vi "Example.vi"() -> ()   [LabVIEW 2014, in "ND2_Reader_32.lvlib"]
uses:
  ND2_Reader_32.lvlib
panel:
  out "Image":T1(plugin-control)
  out "Avg Frame Process Time":dbl
  in  "stop":bool
  out "Frame Timing":u32(graph)
  out "Process Time":dbl
  in  "FilePath":path=path "C:/Users/VirtualUser/Desktop/EPA Image Processing/test images/150806-005.nd2"
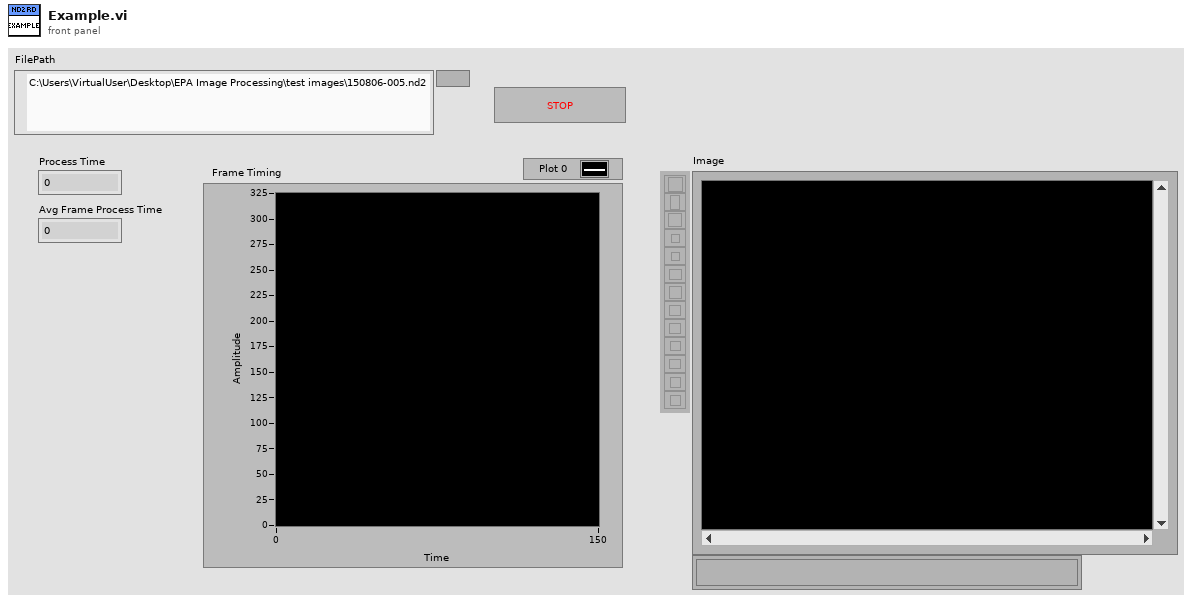
[diagram p1: front panel]
types:
  T1 = typedef "IMAQ Image.ctl" = refnum<image>
  T2 = typedef "cluster_LIMPICTURE.ctl" = cluster{"uiWidth":u32, "uiHeight":u32, "uiBitsPerComp":u32, "uiComponents":u32, "uiWidthBytes":u32, "uiSize":u32, "pImageData":u32}
  T3 = typedef "numeric_LIMFILEHANDLE.ctl" = i32
  T4 = typedef "Image Type" = u32
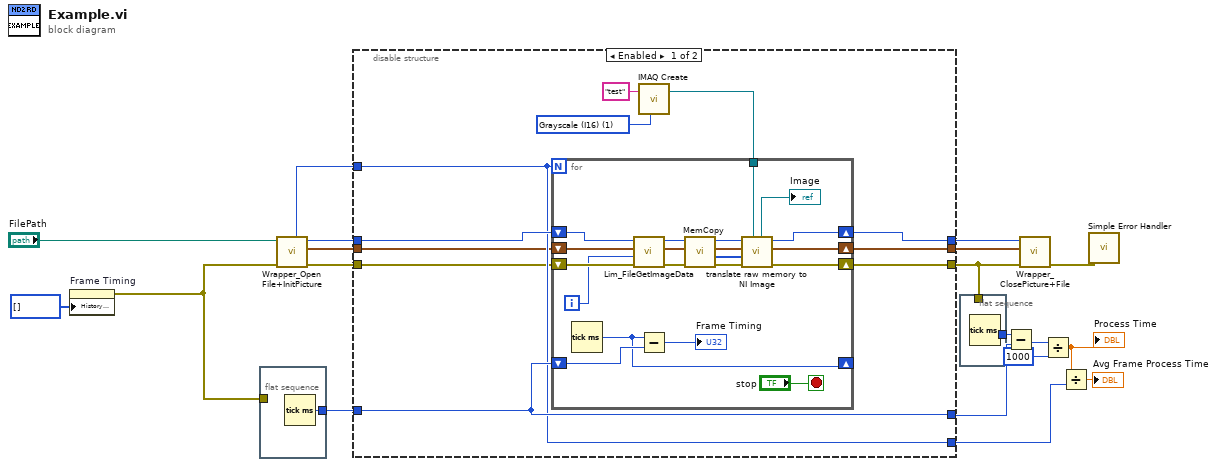
[diagram p0: block diagram]
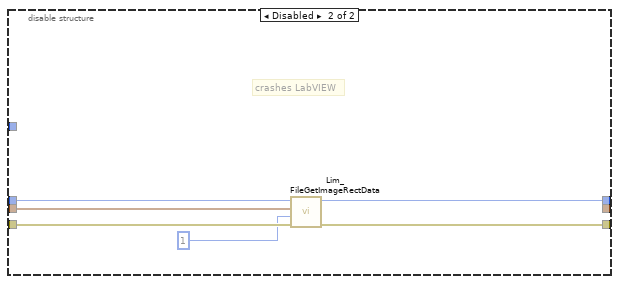
[diagram p2: hidden frame]
diagram:
  n1 = property on="Frame Timing" class="WFChart (strict)"("History Data"=u32[] []) -> (error out=w6:errorcluster)  [unwired: 2 in, 1 out]
  n2 = flat-sequence {
    tunnel: [w20] -> w18
    tunnel: w6 -> [_]
    frame #0 {
      n3 = Tick Count (ms)() -> (millisecond timer value=w20:u32)
    }
  }
  n4 = call "Wrapper_Open File+InitPicture.vi"("error in (no error)"=w6, "FilePath"="FilePath") -> ("error out"=w10:errorcluster, "LIMPICTUREout"=w9:T2, "hFile out"=w8:T3, "N Frames (= uiSequenceCount)"=w5:u32)  [unwired: 6 in]
  n5 = disable-structure shown="Enabled" {
    disable-tunnel: [w22 w55] -> w4
    disable-tunnel: [w23 w56] -> w2
    disable-tunnel: w9 -> [w24 w53]
    disable-tunnel: w8 -> [w27 w57]
    disable-tunnel: w10 -> [w25 w54]
    disable-tunnel: w18 -> [w31 _]
    disable-tunnel: [w31 _] -> w16
    disable-tunnel: [w26 _] -> w12
    disable-tunnel: w5 -> [w26 _]
    disable-tunnel: [w21 _] -> w1
    frame Enabled {
      w29 = T4 1 items=["Grayscale (U8)", "Grayscale (I16)", "Grayscale (SGL)", "Complex (CSG)", "RGB (U32)", "HSL (U32)", "RGB (U64)", "Grayscale (U16)"] ("Image Type")
      n6 = call "IMAQ Create"("Image Name"="test", "Image Type"=w29) -> ("New Image"=w28:T1)  [unwired: 3 in, 1 out]
      n7 = for {
        N: w26 -> [_]
        shift-right: [w43] -> w23
        shift-left: w27 -> [w51]
        shift-right: [w32] -> w21
        shift-left: w24 -> [w50]
        shift-right: [w42] -> w22
        shift-left: w25 -> [w49]
        shift-right: [w46] -> _
        shift-left: w31 -> [w47]
        tunnel: w28 -> [w40]
        i -> [w48]
        stop <- "stop" stop-if-true
        n8 = Tick Count (ms)() -> (millisecond timer value=w46:u32)
        n9 = call "Lim_FileGetImageData.vi"("error in (no error)"=w49, "frameindex"=w48, "LIMPICTURE in"=w50, "hFile in"=w51) -> ("error out"=w45:errorcluster, "LIMPICTURE out"=w33:T2, "hFile out"=w44:T3)  [unwired: 4 in, 1 out]
        n10 = Subtract(x=w46, y=w47) -> (x-y=→"Frame Timing":u32)
        n11 = call "MemCopy.vi"("error in (no error)"=w45, "LIMPICTURE in"=w33, "hFile in"=w44) -> ("error out"=w38:errorcluster, "pBuffer out"=w34:u8[], "LIMPICTURE out"=w35:T2, "hFile out"=w37:T3)  [unwired: 5 in]
        n12 = call "translate raw memory to NI Image.vi"("Image in"=w40, "error in (no error)"=w38, "pBuffer"=w34, "LIMPICTURE in"=w35, "hFile in"=w37) -> ("error out"=w42:errorcluster, "LIMPICTURE out"=w32:T2, "hFile out"=w43:T3, "Image out"=→"Image":T1)  [unwired: 3 in]
      }
    }
    frame Disabled {
      # "crashes LabVIEW"
      n13 = call "Lim_FileGetImageRectData.vi"("error in (no error)"=w54, "frameindex"=u32 1, "LIMATTRIBUTES"=w53, "hFile in"=w57) -> ("error out"=w55:errorcluster, "hFile out"=w56:T3)  [unwired: 5 in, 1 out]
    }
  }
  n14 = flat-sequence {
    tunnel: [w58] -> w17
    tunnel: w4 -> [_]
    frame #0 {
      n15 = Tick Count (ms)() -> (millisecond timer value=w58:u32)
    }
  }
  n16 = Subtract(x=w17, y=w16) -> (x-y=w15:u32)
  n17 = call "Wrapper_ClosePicture+File.vi"("error in (no error)"=w4, "LIMPICTURE"=w1, "hFile in"=w2) -> ("error out"=w3:errorcluster)  [unwired: 8 in]
  n18 = Divide(x=w15, y=u32 1000) -> (x/y=w13:dbl)
  "Process Time" <- w13
  n19 = Divide(x=w13, y=w12) -> (x/y=→"Avg Frame Process Time":dbl)
  n20 = call <vilib>:"Simple Error Handler.vi"("error in (no error)"=w3) -> ()  [unwired: 4 in, 5 out]
